vi "SAOMM-ROIEnums.vi"(7 "Path":path) -> (8 "StringEnums":string[](array[string]), 13 "ROISizes":i32[](array[numeric]))   [LabVIEW 2011]
uses:
  <vilib>/Utility/config.llb/Read Key (Double).vi
  <vilib>/Utility/config.llb/Read Key (String).vi
  <vilib>/Utility/config.llb/NI_LVConfig.lvlib
panel:
  out "array":dbl[](array[numeric])
  out "value":string
  out "PixScale1":dbl
  out "PixScale2":dbl
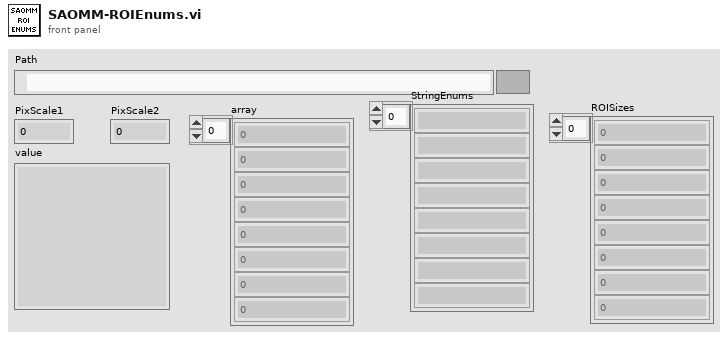
[diagram p1: front panel]
types:
  T1 = typedef "NI_LVConfig.lvlib/Config Data RefNum.ctl" = refnum<k1>
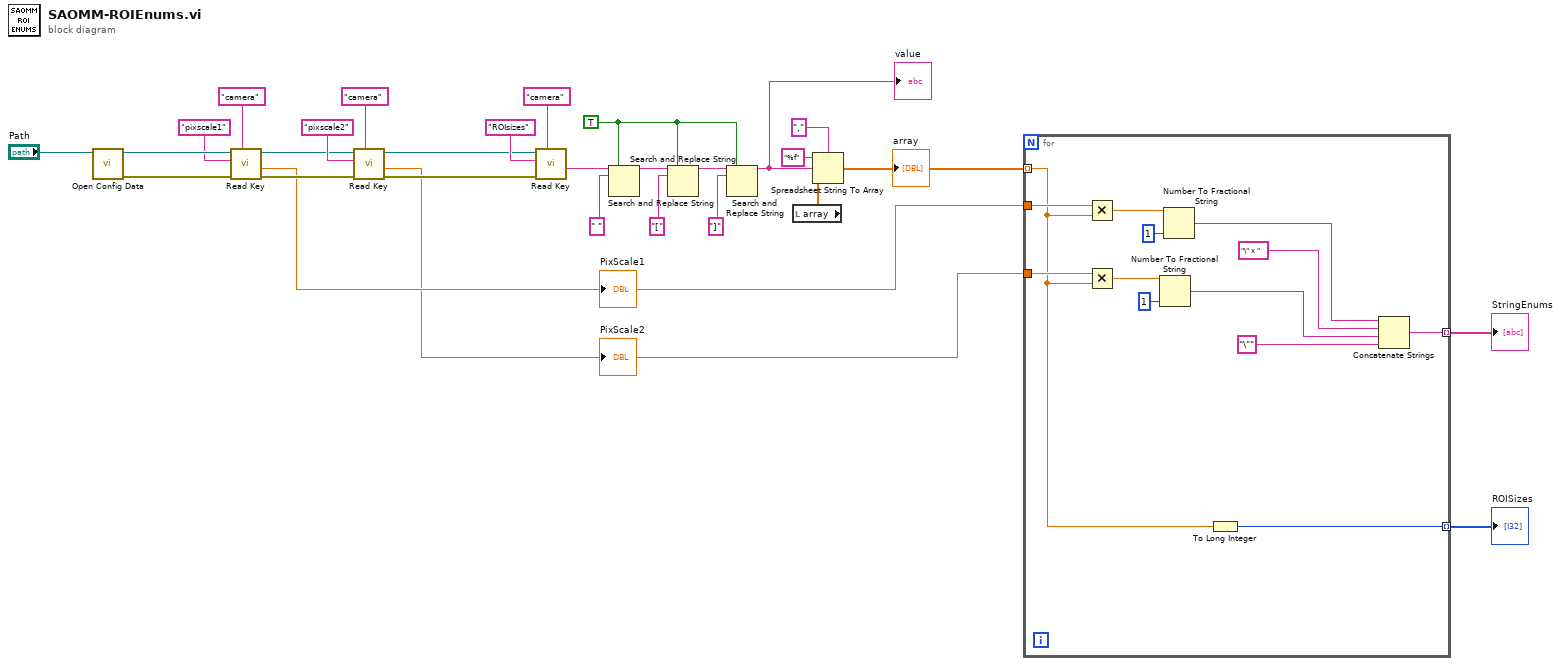
[diagram p0: block diagram]
diagram:
  w12 = TRUE ("replace all? (F)")
  n1 = call <vilib>:"Open Config Data.vi"("configuration file path"="Path") -> ("error out"=w25:errorcluster, "refnum"=w26:T1)  [unwired: 8 in, 1 out]
  n2 = call-poly <vilib>:"Read Key.vi"("section"="camera", "error in (no error)"=w25, "key"="pixscale1" ("section"), "refnum"=w26) -> ("error out"=w19:errorcluster, "value"=w4:dbl, "refnum out"=w20:T1)  [unwired: 4 in, 1 out]
  "PixScale1" <- w4
  n3 = call-poly <vilib>:"Read Key.vi"("section"="camera", "error in (no error)"=w19, "key"="pixscale2" ("section"), "refnum"=w20) -> ("error out"=w17:errorcluster, "value"=w3:dbl, "refnum out"=w18:T1)  [unwired: 4 in, 1 out]
  "PixScale2" <- w3
  n4 = call-poly <vilib>:"Read Key.vi"("section"="camera", "error in (no error)"=w17, "key"="ROIsizes" ("section"), "refnum"=w18) -> ("value"=w16:string)  [unwired: 4 in, 3 out]
  n5 = Search and Replace String(replace all?=w12, input string=w16, search string=" ") -> (result string=w14:string)  [unwired: 5 in, 3 out]
  n6 = Search and Replace String(replace all?=w12, input string=w14, search string="[") -> (result string=w13:string)  [unwired: 5 in, 3 out]
  n7 = Search and Replace String(replace all?=w12, input string=w13, search string="]") -> (result string=w7:string)  [unwired: 5 in, 3 out]
  "value" <- w7
  n8 = local read "array"() -> (w6:dbl[])
  n9 = Spreadsheet String To Array(delimiter (Tab)=",", format string="%f", spreadsheet string=w7, array type (2D Dbl)=w6) -> (array=w5:dbl[])
  "array" <- w5
  n10 = for {
    tunnel: w5 -> [w31] mode=indexing
    tunnel: w4 -> [w37]
    tunnel: w3 -> [w36]
    tunnel: [w32] -> w2 mode=indexing
    tunnel: [w30] -> w1 mode=indexing
    n11 = Multiply(x=w37, y=w31) -> (x*y=w38:dbl)
    n12 = Multiply(x=w36, y=w31) -> (x*y=w39:dbl)
    n13 = Number To Fractional String(number=w39, precision (6)=i16 1) -> (F-format string=w35:string)  [unwired: 2 in]
    n14 = Number To Fractional String(number=w38, precision (6)=i16 1) -> (F-format string=w33:string)  [unwired: 2 in]
    n15 = To Long Integer(number=w31) -> (32bit integer=w30:i32)
    n16 = Concatenate Strings(w33, "\" x ", w35, "\"") -> (w32:string)
  }
  "StringEnums" <- w2
  "ROISizes" <- w1
